vi "adamread.vi"(0 "TCP Connection Refnum in":refnum<k5>, 5 "Modbus Command":T1={"Function Code"=3, "Starting Address"=0, "Quantity"=8, "Data"=[], "Discrete"=[]} {"Function Code" items=["Read Coils"=1, "Read Discrete Inputs"=2, "Read Holding Registers"=3, "Read Input Registers"=4, "Write Single Coil"=5, "Write Single Register"=6, "Read Exception Status"=7, "Write Multiple Coils"=15, "Write Multiple Registers"=16]}, 11 "error in (no error)":errorcluster, 12 "timout":u32) -> (4 "TCP Connection Refnum (dup)":refnum<k5>, 10 "Slave Input Registers 2":dbl[](array[numeric]) caption="Slave Input Registers (Read Only)", 15 "error out 2":errorcluster)   [LabVIEW 2019]
uses:
  NI Modbus.llb/MB Modbus Command.ctl
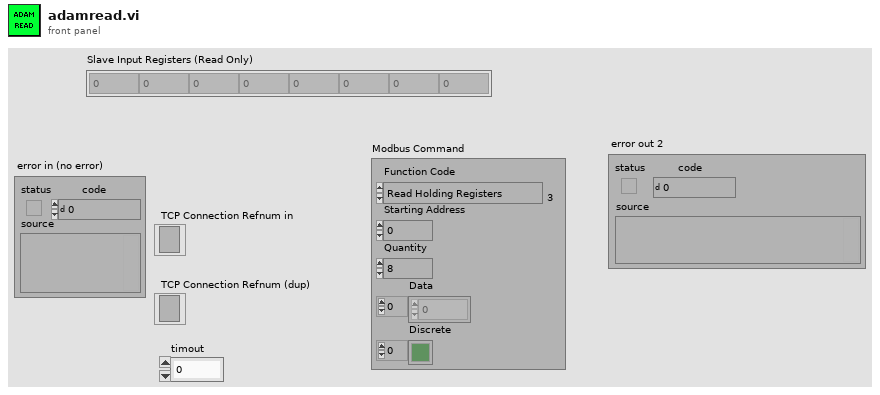
[diagram p1: front panel]
types:
  T1 = typedef "MB Modbus Command.ctl" = cluster{"Function Code":u8, "Starting Address":u16, "Quantity":u16, "Data":u16[], "Discrete":bool[]}
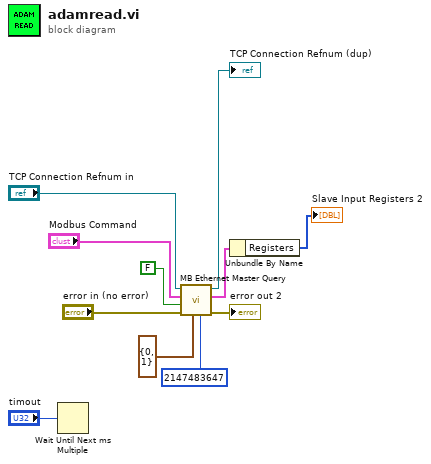
[diagram p0: block diagram]
diagram:
  n1 = Wait Until Next ms Multiple(millisecond multiple="timout") -> ()  [unwired: 1 out]
  n2 = call "MB Ethernet Master Query.vi"("Timeout"=2147483647, "MBAP Header"=cluster{"Transaction ID":u16, "Unit ID":u8} {"Transaction ID"=0, "Unit ID"=1}, "error in (no error)"="error in (no error)", "Use MODBUS Data Unit?"=FALSE, "Modbus Command"="Modbus Command", "TCP Connection Refnum in"="TCP Connection Refnum in") -> ("error out"=→"error out 2":errorcluster, "Registers"=w7:cluster{"Registers":u16[], "Discrete":bool[]}, "TCP Connection Refnum (dup)"=→"TCP Connection Refnum (dup)":refnum<k5>)  [unwired: 1 in, 2 out]
  n3 = Unbundle By Name(w7) -> ("Registers"=→"Slave Input Registers 2":u16[])
